vi "Open Test Case.vi"(8 "error in (no error)":errorcluster, 10 "Tag":string, 11 "Test Finder In":refnum<class "Test Finder.lvclass">) -> (0 "error out":errorcluster, 1 "VI name valid?":bool, 3 "Test Finder Out":refnum<class "Test Finder.lvclass">)   [LabVIEW 2020, in "Test Finder.lvclass"]
uses:
  Test Finder.lvclass
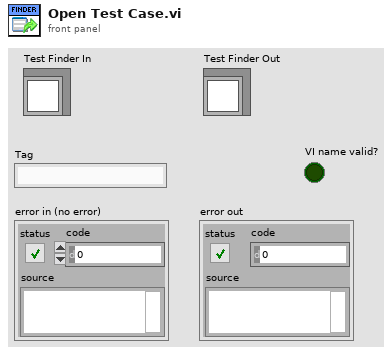
[diagram p1: front panel]
types:
  T1 = enum32{"Invalid", "Standard", "Closed", "Hidden", "Minimized", "Maximized"}
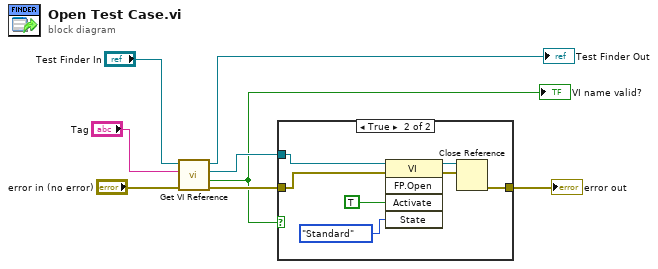
[diagram p0: block diagram]
diagram:
  n1 = call "Get VI Reference.vi"("error in (no error)"="error in (no error)", "VI name"="Tag", "Test Finder"="Test Finder In") -> ("error out"=w6:errorcluster, "Found?"=w1:bool, "Reference"=w5:refnum<vi>, "Test Finder out"=→"Test Finder Out":refnum<class "Test Finder.lvclass">)  [unwired: 5 in]
  "VI name valid?" <- w1
  n2 = case shown="True" w1 {
    tunnel: [w9 w12] -> w7
    tunnel: w6 -> [w9 w11]
    tunnel: w5 -> [_ w10]
    frame False {
    }
    frame True {
      n3 = invoke class="VI" method="FP.Open"(reference=w10, error in=w11, "Activate"=TRUE ("Activate?"), "State"=T1."Standard") -> (reference out=w13:refnum<vi>, error out=w14:errorcluster)  [unwired: 1 in, 3 out]
      n4 = Close Reference(reference=w13, error in (no error)=w14) -> (error out=w12:errorcluster)
    }
  }
  "error out" <- w7
